vi "Disconnect PC Beamage.vi"(8 "error in":errorcluster) -> (0 "error out":errorcluster, 1 "Disconnected":bool)   [LabVIEW 2009]
uses:
  BeamageNP.dll
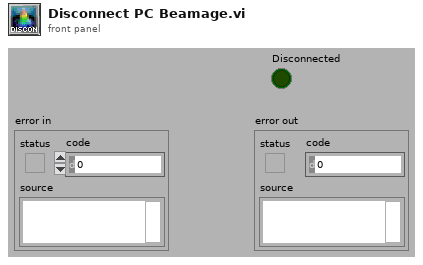
[diagram p1: front panel]
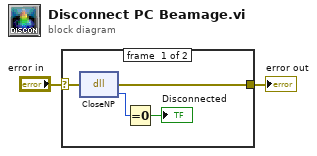
[diagram p0: block diagram]
diagram:
  n1 = case shown="No Error" "error in" {
    selector: "error in" -> [w5 w7]
    tunnel: [w4 w7] -> w1
    frame #0 {
      n2 = dll-call lib="S:/LabView Files/Beamage 3.0/BeamageNP.dll" fn="CloseNP"(error in=w5) -> (error out=w4:errorcluster, "return type"=w3:i32)  [unwired: 2 in, 1 out]
      n3 = Equal To 0?(x=w3) -> (x = 0?=→"Disconnected":bool)
    }
    frame #1 {
    }
  }
  "error out" <- w1
